vi "Axes Order.vi"(0 "string":string[](array[string])) -> ()   [LabVIEW 2021]
uses:
  A3200.lvclass
panel:
  out "A3200.lvclass":refnum<class "A3200.lvclass">
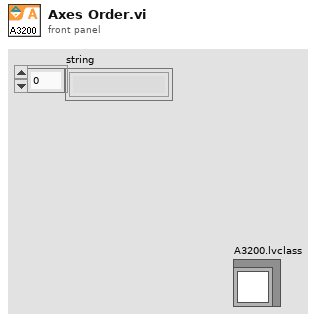
[diagram p1: front panel]
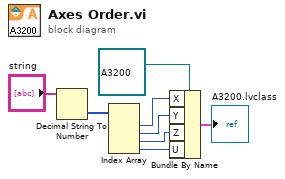
[diagram p0: block diagram]
diagram:
  n1 = Decimal String To Number(string="string") -> (number=w2:i32[])  [unwired: 2 in, 1 out]
  n2 = Index Array(array=w2) -> (element #1=w6:i32, element #2=w5:i32, element #3=w4:i32, element #4=w3:i32)  [unwired: 4 in]
  n3 = Bundle By Name(cluster=refnum<class "A3200.lvclass"> refnum ("A3200.lvclass"), "X"=w6, "Y"=w5, "Z"=w4, "U"=w3) -> (→"A3200.lvclass":cluster{})
